vi "Rotate.vi"(8 "error in (no error)":errorcluster, 10 "Direction":bool, 11 "StepperController in":refnum<class "StepperController.lvclass">) -> (0 "error out":errorcluster, 1 "NewPosition":dbl, 2 "DidMove":bool, 3 "StepperController out":refnum<class "StepperController.lvclass">, 4 "AmountMoved":dbl)   [LabVIEW 2013, in "StepperController.lvclass"]
uses:
  StepperController.lvclass
  StepperController.lvclass/StepperController.ctl
  <vilib>/DAQmx/write.llb/DAQmx Write (Digital Bool 1Line 1Point).vi
  <vilib>/DAQmx/miscellaneous.llb/DAQmx Fill In Error Info.vi
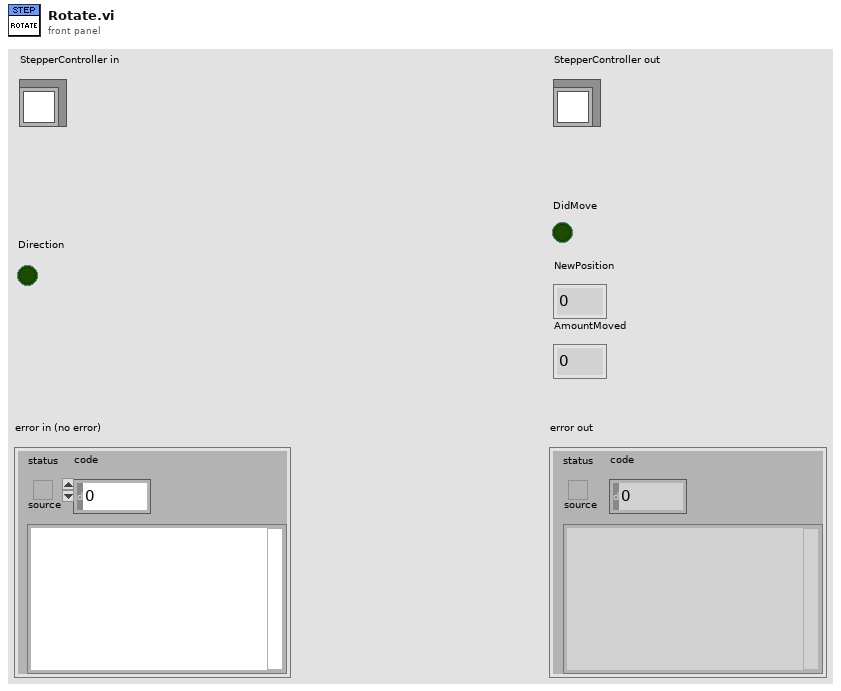
[diagram p1: front panel]
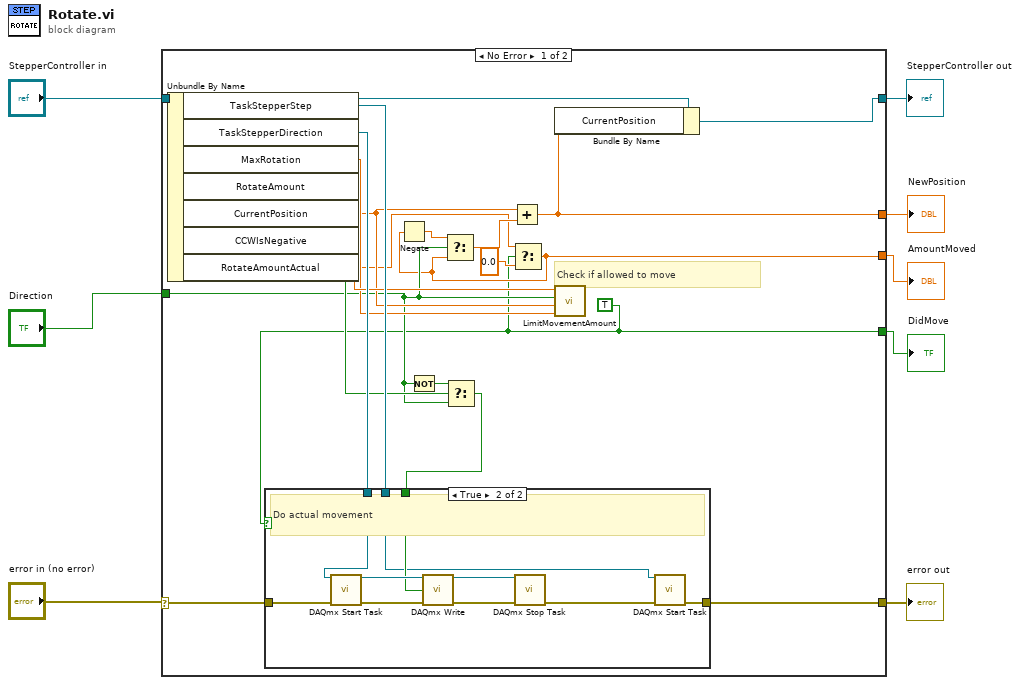
[diagram p0: block diagram]
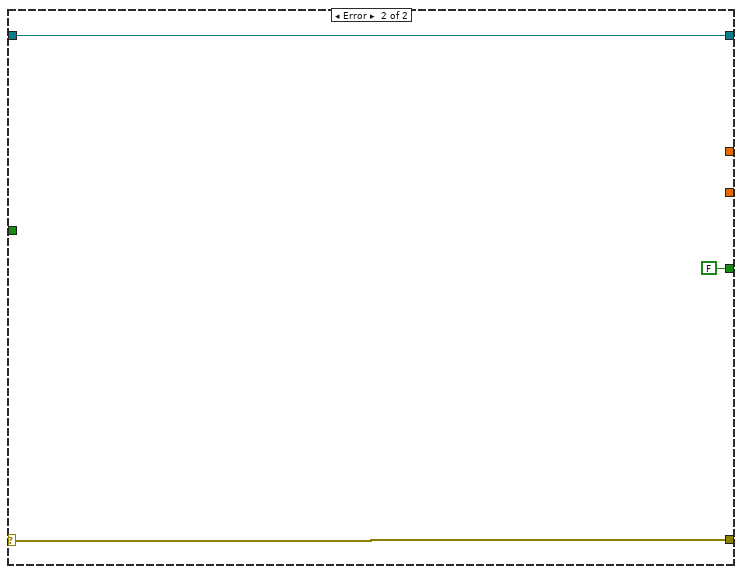
[diagram p3: hidden frame]
diagram:
  n1 = case shown="No Error" "error in (no error)" {
    selector: "error in (no error)" -> [w27 w42]
    tunnel: [w26 w42] -> w7
    tunnel: "StepperController in" -> [w22 w41]
    tunnel: [w20 w41] -> w5
    tunnel: [w9 FALSE ("Movement allowed")] -> w1
    tunnel: "Direction" -> [w15 _]
    tunnel: [w16 _] -> w3
    tunnel: [w10 _] -> w2
    frame No Error {
      w9 = TRUE
      # "Check if allowed to move"
      n2 = Unbundle By Name(w22) -> ("TaskStepperStep"=w28:refnum<k21>, "TaskStepperDirection"=w25:refnum<k21>, "MaxRotation"=w23:dbl, "RotateAmount"=w24:dbl, "CurrentPosition"=w21:dbl, "CCWIsNegative"=w17:bool, "RotateAmountActual"=w12:dbl)
      n3 = Not(x=w15) -> (.not. x?=w19:bool)
      n4 = Select(t=w19, s=w17, f=w15) -> (s? t:f=w18:bool)
      n5 = case shown="True" w9 {
        tunnel: w28 -> [_ w31]
        tunnel: w27 -> [w29 w34]
        tunnel: [w29 w33] -> w26
        tunnel: w25 -> [_ w30]
        tunnel: w18 -> [_ w32]
        frame False {
        }
        frame True {
          # "Do actual movement"
          n6 = call <vilib>:"DAQmx Start Task.vi"("task/channels in"=w30, "error in"=w34) -> ("task out"=w39:refnum<k21>, "error out"=w38:errorcluster)  [unwired: 12 in]
          n7 = call-poly <vilib>:"DAQmx Write.vi"("task/channels in"=w39, "data"=w32, "error in"=w38) -> ("task out"=w37:refnum<k21>, "error out"=w36:errorcluster)  [unwired: 10 in, 1 out]
          n8 = call <vilib>:"DAQmx Stop Task.vi"("task/channels in"=w37, "error in"=w36) -> ("error out"=w35:errorcluster)  [unwired: 12 in, 1 out]
          n9 = call <vilib>:"DAQmx Start Task.vi"("task/channels in"=w31, "error in"=w35) -> ("error out"=w33:errorcluster)  [unwired: 12 in, 1 out]
        }
      }
      n10 = Select(t=w12, s=w9, f=0.0) -> (s? t:f=w10:dbl)
      n11 = Negate(x=w10) -> (-x=w13:dbl)
      n12 = Select(t=w13, s=w15, f=w10) -> (s? t:f=w14:dbl)
      n13 = Add(x=w21, y=w14) -> (x+y=w16:dbl)
      n14 = Bundle By Name(cluster=w22, "CurrentPosition"=w16) -> (w20:refnum<class "StepperController.lvclass">)
      n15 = call "LimitMovementAmount.vi"("Max rotation"=w23, "Current position"=w21, "Direction"=w15, "Move amount in"=w24) -> ()  [unwired: 6 in, 2 out]
    }
    frame Error {
    }
  }
  "StepperController out" <- w5
  "error out" <- w7
  "DidMove" <- w1
  "NewPosition" <- w3
  "AmountMoved" <- w2
